vi "PathPlanner_Waypoint_Flip.vi"(11 "Waypoint":T1 {"nextControl"."Y" format="%14.3f"; "nextControl"."X" format="%14.3f"; "anchor"."Y" format="%14.3f"; "anchor"."X" format="%14.3f"; "prevControl"."Y" format="%14.3f"; "prevControl"."X" format="%14.3f"}) -> (3 "FlippedWaypoint":T1 {"nextControl"."Y" format="%14.3f"; "nextControl"."X" format="%14.3f"; "anchor"."Y" format="%14.3f"; "anchor"."X" format="%14.3f"; "prevControl"."Y" format="%14.3f"; "prevControl"."X" format="%14.3f"})   [LabVIEW 2019, in "PathPlanner24.lvlib"]
doc: "Flip this waypoint to the other side of the field, maintaining a blue alliance origin\n\nInputs: \n - Waypoint - cluster - The waypoint to flip\n\nOutputs:\n - FlippedWaypoint - cluster - The flipped waypoint"
uses:
  PathPlanner24.lvlib
  TypeDef/PathPlannerWaypoint.ctl
  <vilib>/Rock Robotics/WPI/ThirdParty/JAS_Junk/TrajLib/TypeDef/TRANSLATION2D.ctl
  PathPlanner_FieldUtil_SymmetryType.vi
  PathPlanner_FieldUtil_FieldSizeY.vi
  <vilib>/Rock Robotics/WPI/ThirdParty/JAS_Junk/TrajLib/Translation2d_GetXY.vi
  <vilib>/Rock Robotics/WPI/ThirdParty/JAS_Junk/TrajLib/Translation2d_Create.vi
  PathPlanner_FieldUtil_FieldSizeX.vi
  <vilib>/Rock Robotics/WPI/ThirdParty/JAS_Junk/TrajLib/Conv_Feet_Meters.vi
  <vilib>/Rock Robotics/WPI/ThirdParty/JAS_Junk/TrajLib/Trajectory_Library.lvlib
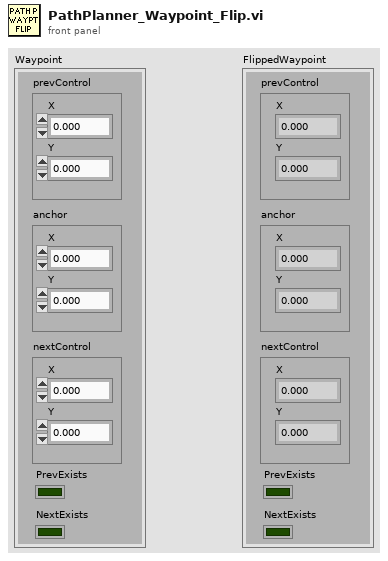
[diagram p1: front panel]
types:
  T1 = typedef "PathPlanner24.lvlib/PathPlannerWaypoint.ctl" = cluster{"prevControl":T2, "anchor":T2, "nextControl":T2, "PrevExists":bool, "NextExists":bool}
  T2 = typedef "Trajectory_Library.lvlib/TRANSLATION2D.ctl" = cluster{"X":dbl, "Y":dbl}
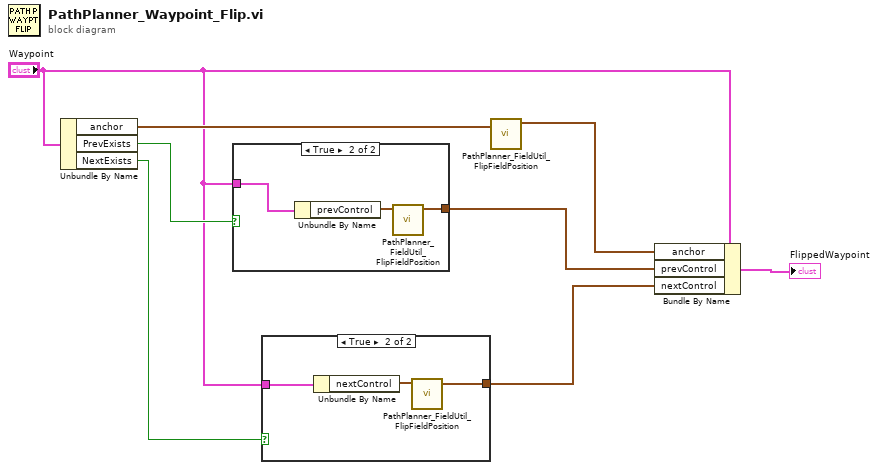
[diagram p0: block diagram]
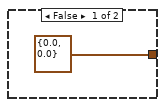
[diagram p2: hidden frame]
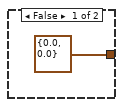
[diagram p3: hidden frame]
diagram:
  n1 = Unbundle By Name("Waypoint") -> ("anchor"=w3:T2, "PrevExists"=w5:bool, "NextExists"=w4:bool)
  n2 = case shown="True" w5 {
    tunnel: [T2 {"X"=0.0, "Y"=0.0} ("prevControl") w11] -> w7
    tunnel: "Waypoint" -> [_ w10]
    frame False {
    }
    frame True {
      n3 = Unbundle By Name(w10) -> ("prevControl"=w12:T2)
      n4 = call "PathPlanner_FieldUtil_FlipFieldPosition.vi"("FieldPosition"=w12) -> ("FlippedFieldPosition"=w11:T2)  [unwired: 10 in]
    }
  }
  n5 = case shown="True" w4 {
    tunnel: [T2 {"X"=0.0, "Y"=0.0} ("prevControl") w15] -> w6
    tunnel: "Waypoint" -> [_ w14]
    frame False {
    }
    frame True {
      n6 = Unbundle By Name(w14) -> ("nextControl"=w16:T2)
      n7 = call "PathPlanner_FieldUtil_FlipFieldPosition.vi"("FieldPosition"=w16) -> ("FlippedFieldPosition"=w15:T2)  [unwired: 10 in]
    }
  }
  n8 = call "PathPlanner_FieldUtil_FlipFieldPosition.vi"("FieldPosition"=w3) -> ("FlippedFieldPosition"=w2:T2)  [unwired: 10 in]
  n9 = Bundle By Name(cluster="Waypoint", "anchor"=w2, "prevControl"=w7, "nextControl"=w6) -> (→"FlippedWaypoint":T1)
